vi "RunSimulationBattery-Media.vi"() -> ()   [LabVIEW 2019]
panel:
  in  "File Prefix":string="BigSlab"
  out "Percent Complete":dbl(slide) scale=0.0..1.0
  in  "Anisotropy G":dbl[](array[numeric])=[0.92]
  in  "Scattering Coefficient":dbl[](array[numeric])=[0.0, 0.1, 0.177827941, 0.316227766, 0.562341325, 1.0, 1.77827941, 3.16227766, 5.623413252, 10.0]
  in  "Use Slab Geometry (F: Sphere)":bool
  out "Time to End":cluster{"Time To End":dbl, "unit":string} {"Time To End" format="%#_4g"}
  in  "Depths (mm)":dbl[](array[numeric])=[1e-09, 0.1, 0.2, 0.3, 0.4, 0.5, 0.6, 0.7, 0.8, 0.9, 1.0, 1.1, 1.2, 1.3, 1.4, 1.5, 1.6, 1.7, 1.8, 1.9, 2.0, 2.5, 3.0, 3.5, 4.0, 4.5, 5.0] format="%#_10g"
  in  "Folder":path=path "D:/Ian_s Dropbox/Dropbox/PostDoc/Programs/Data/2020-01-08 BigSlab"
  in  "N Photons":i32=300000
  in  "Simulation Grain (mm)":dbl=0.0001
  in  "Radius (mm)":dbl=5.0
  # "1 pm = 1E-9 mm"
  # "0.1\n0.177827941\n0.316227766\n0.562341325\n1\n1.77827941\n3.16227766\n5.623413252\n10"
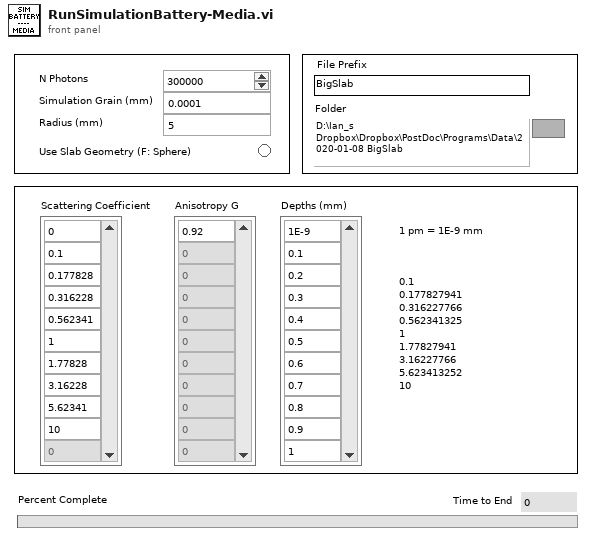
[diagram p1: front panel]
types:
  T1 = cluster{"Scattering Coefficient":dbl[], "Interleave?":bool}
  T2 = cluster{"Anisotropy G":dbl[], "Interleave?":bool}
  T3 = cluster{"Depths (mm)":dbl[], "Interleave?":bool}[]
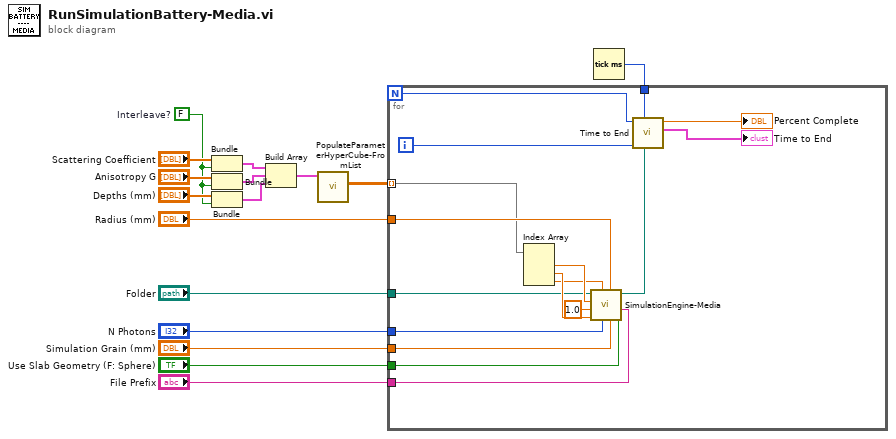
[diagram p0: block diagram]
diagram:
  w1 = FALSE  # Interleave?
  n1 = Bundle("Scattering Coefficient"="Scattering Coefficient", "Interleave?"=w1) -> (w6:T1)  [unwired: 1 in]
  n2 = Bundle("Anisotropy G"="Anisotropy G", "Interleave?"=w1) -> (w7:T2)  [unwired: 1 in]
  n3 = Bundle("Depths (mm)"="Depths (mm)", "Interleave?"=w1) -> (w8:cluster{"Depths (mm)":dbl[], "Interleave?":bool})  [unwired: 1 in]
  n4 = Build Array(w6, w7, w8) -> (w5:T3)
  n5 = call "PopulateParameterHyperCube-FromList.vi"("Range and Resolution Preview"=w5) -> ("2D Array"=w11:dbl[][])  [unwired: 8 in, 2 out]
  n6 = Tick Count (ms)() -> (millisecond timer value=w10:u32)
  n7 = for {
    N -> [w20]
    tunnel: "Folder" -> [w24]
    tunnel: "Radius (mm)" -> [w33]
    tunnel: "Simulation Grain (mm)" -> [w32]
    tunnel: "N Photons" -> [w31]
    tunnel: "Use Slab Geometry (F: Sphere)" -> [w30]
    tunnel: w11 -> [w29] mode=indexing
    tunnel: w10 -> [w21]
    tunnel: "File Prefix" -> [w25]
    i -> [w18]
    n8 = Index Array(array=w29) -> (element #1=w28:dbl, element #2=w27:dbl, element #3=w26:dbl)  [unwired: 3 in]
    n9 = call "SimulationEngine-Media.vi"("Use Slab Geometry (F: Sphere)"=w30, "File Prefix"=w25, "Simulation Grain (mm)"=w32, "Radius (mm)"=w33, "N Photons"=w31, "Starting Depth (mm)"=w26, "G"=w27, "Absorption Coefficient"=1.0, "Scattering Coefficient"=w28, "folder path"=w24) -> ("new file path (Not A Path if cancelled)"=w19:path)  [unwired: 1 out]
    n10 = call "Time to End.vi"("Trigger"=w19, "Start Time (ms)"=w21, "i"=w18, "N"=w20) -> ("Time to End"=→"Time to End":cluster{"Time To End":dbl, "unit":string}, "Percent Complete"=→"Percent Complete":dbl)  [unwired: 3 in, 3 out]
  }
